vi "Analyse BMP.vi"(0 "Chemin d'acces":path, 5 "Lec Fic Midi":bool) -> (4 "Resultat Lecture":string, 6 "Matrix":u8[](array[numeric]))   [LabVIEW 2014]
panel:
  out "Pixel :":u8[](array[numeric])
  out "Palette :":T1(array[cluster])
  out "Offset pixel":u32
  # "Entrées :"
  # "Sorties :"
  # "Variables internes :"
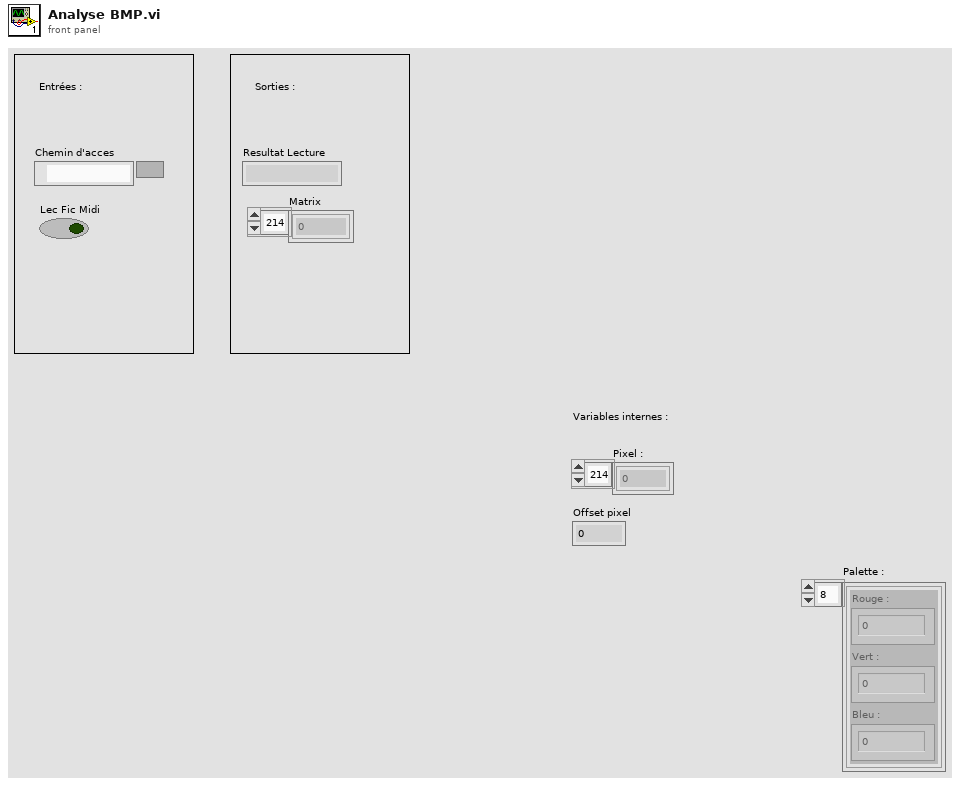
[diagram p1: front panel]
types:
  T1 = cluster{"Rouge : ":u8, "Vert :":u8, "Bleu :":u8}[]
  T2 = enum16{"open", "replace", "create", "open or create", "replace or create", "replace or create with confirmation"}
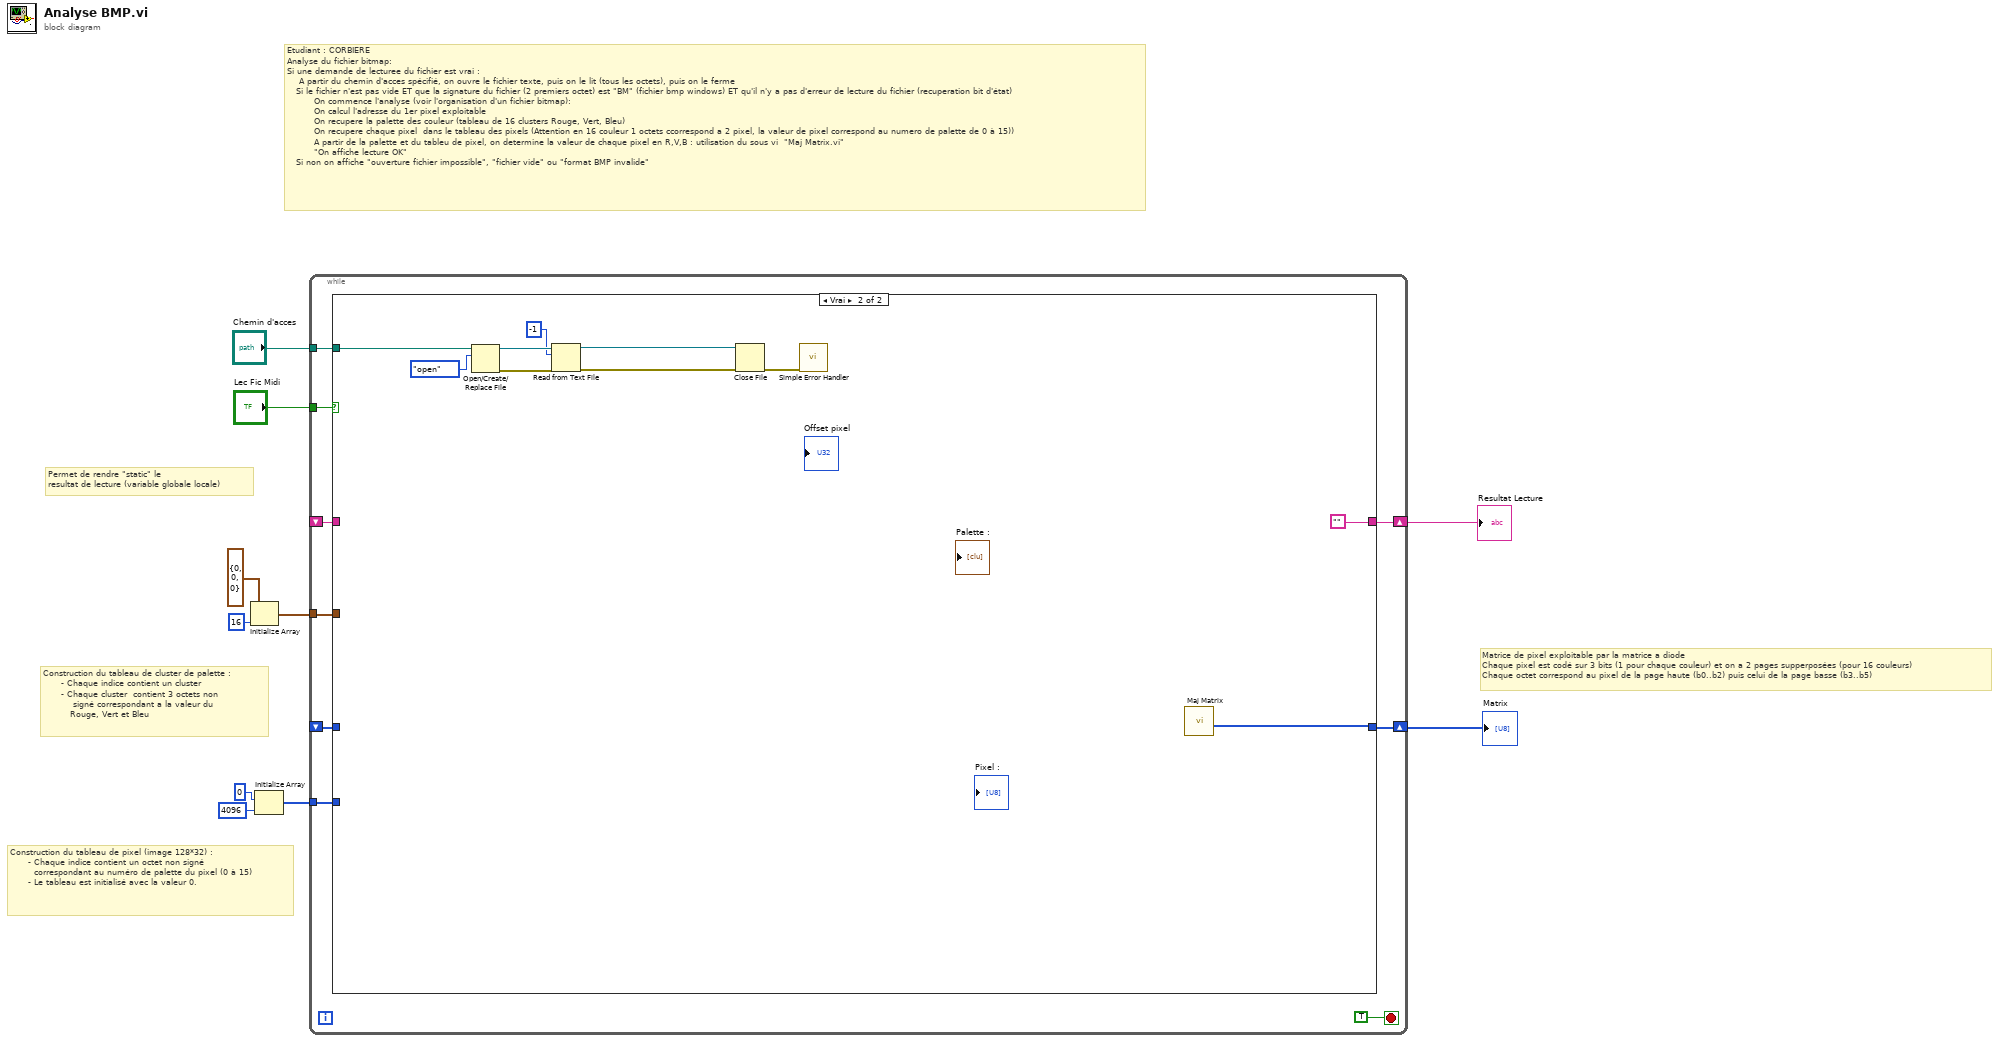
[diagram p0: block diagram]
diagram:
  # "Permet de rendre \"static\" le \nresultat de lecture (variable globale locale)"
  # "Matrice de pixel exploitable par la matrice a diode\nChaque pixel est codé sur 3 bits (1 pour chaque couleur) et on a 2 pages supperposées (pour 16 couleurs)\nChaque octet correspond au pixel de la page haute (b0..b2) puis celui de la page basse (b3..b5)"
  # "Construction du tableau de pixel (image 128*32) :\n      - Chaque indice contient un octet non signé\n        correspondant au numéro de palette du pixel (0 à 15)\n      - Le tableau est initialisé avec la valeur 0."
  # "Construction du tableau de cluster de palette :\n      - Chaque indice contient un cluster\n      - Chaque cluster  contient 3 octets non\n          signé correspondant a la valeur du\n         Rouge, Vert et Bleu"
  # "Etudiant : CORBIERE\nAnalyse du fichier bitmap:\nSi une demande de lecturee du fichier est vrai :\n    A partir du chemin d'acces spécifié, on ouvre le fichier texte, puis on le lit (tous les octets), puis on le ferme \n   Si le fichier n'est pas vide ET que la signature du fichier (2 premiers octet) est \"BM\" (fichier bmp windows) ET qu'il n'y a pas d'erreur de lecture du fichier (recuperation bit d'état)\n         On commence l'analyse (voir l'organisation d'un fichier bitmap): \n         On calcul l'adresse du 1er pixel exploitable\n         On recupere la palette des couleur (tableau de 16 clusters Rouge, Vert, Bleu)\n         On recupere chaque pixel  dans le tableau des pixels (Attention en 16 couleur 1 octets ccorrespond a 2 pixel, la valeur de pixel correspond au numero de palette de 0 à 15))\n         A partir de la palette et du tableu de pixel, on determine la valeur de chaque pixel en R,V,B : utilisation du sous vi  \"Maj Matrix.vi\"\n         \"On affiche lecture OK\"\n   Si non on affiche \"ouverture fichier impossible\", \"fichier vide\" ou \"format BMP invalide\""
  n1 = Initialize Array(cluster{"Rouge : ":u8, "Vert :":u8, "Bleu :":u8} {"Rouge : "=0, "Vert :"=0, "Bleu :"=0} ("Pixel :"), 16) -> (w6:T1)
  n2 = Initialize Array(u8 0, 4096) -> (w3:u8[])
  n3 = while {
    tunnel: "Chemin d'acces" -> [w19]
    tunnel: "Lec Fic Midi" -> [w18]
    shift-right: [w16] -> w1
    shift-left: _ -> [w15]
    tunnel: w3 -> [w13]
    shift-right: [w12] -> w2
    shift-left: _ -> [w11]
    tunnel: w6 -> [w14]
    stop <- TRUE stop-if-true
    n4 = case shown="Vrai" w18 {
      tunnel: w19 -> [_ w26]
      tunnel: [w21 ""] -> w16
      tunnel: w15 -> [w21 _]
      tunnel: w14 -> [_ _]
      tunnel: w13 -> [_ _]
      tunnel: [w20 w23] -> w12
      tunnel: w11 -> [w20 _]
      frame False {
      }
      frame True {
        n5 = Open/Create/Replace File(file path (use dialog)=w26, operation (0:open)=T2."open") -> (refnum out=w31:refnum<file>, error out=w30:errorcluster)  [unwired: 4 in, 1 out]
        n6 = Read from Text File(file (use dialog)=w31, count=-1, error in=w30) -> (refnum out=w29:refnum<file>, error out=w24:errorcluster)  [unwired: 1 in, 2 out]
        n7 = Close File(refnum=w29, error in=w24) -> (error out=w25:errorcluster)  [unwired: 1 out]
        n8 = call <vilib>:"Simple Error Handler.vi"("error in (no error)"=w25) -> ()  [unwired: 4 in, 5 out]
        n9 = call "Maj Matrix.vi"() -> ("Matrix"=w23:u8[])  [unwired: 11 in]
      }
    }
  }
  "Resultat Lecture" <- w1
  "Matrix" <- w2
